vi "HasBuiltInDescription.vi"(4 "Error/warning code":i32) -> (1 "Has built-in description?":bool)   [LabVIEW 2017, in "GPError.lvlib"]
doc: "<B>Has built-in description?</B> will be True only if a description for <B>Error/warning code</B> is known by LabVIEW.\n\nSteen Schmidt\nGPower\n16/11 2012"
uses:
  GPError.lvlib
panel:
  # "Copyright © 2013\nSteen Schmidt, GPower\nSee enclosed license file for terms and conditions"
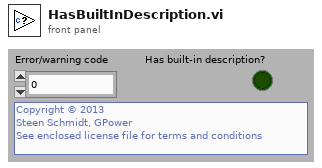
[diagram p1: front panel]
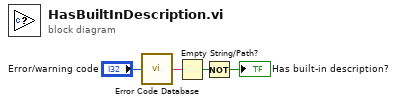
[diagram p0: block diagram]
diagram:
  n1 = call <vilib>:"Error Code Database.vi"("Error Code"="Error/warning code") -> ("Error Text"=w3:string)
  n2 = Empty String/Path?(string/path=w3) -> (empty?=w2:bool)
  n3 = Not(x=w2) -> (.not. x?=→"Has built-in description?":bool)
